vi "TP5.vi"() -> ()   [LabVIEW 2017]
panel:
  out "Boolean 3":bool
  out "Boolean 2":bool
  out "Boolean":bool
  in  "10s":bool
  in  "Tab Control 2":enum32{"Page 1"}(tab)
  in  "Tab Control":enum32{"Page 1"}(tab)
  in  "stop":bool
  in  "pause":bool
  in  "Minuterie":u32 format="%<%M:%S>t"
  in  "rotation":bool
  in  "1m":bool
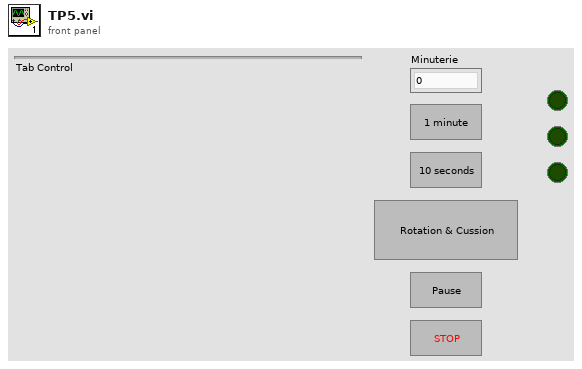
[diagram p1: front panel]
types:
  T1 = enum16{"initialisation", "Mise en marche et vérification", "Cussion", "Pause", "Stop"}
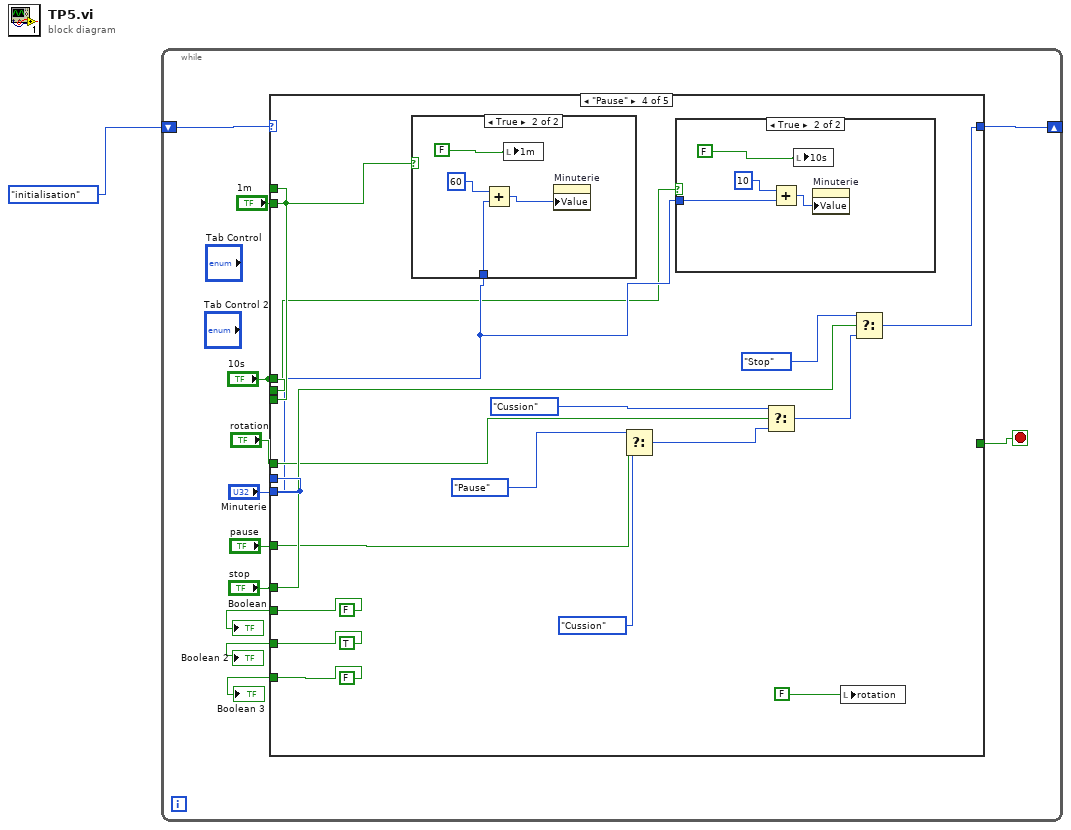
[diagram p0: block diagram]
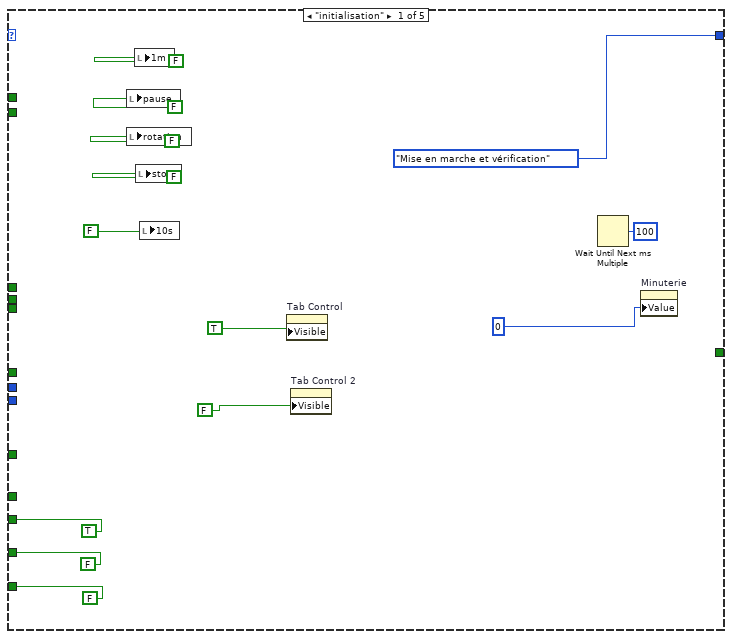
[diagram p2: hidden frame]
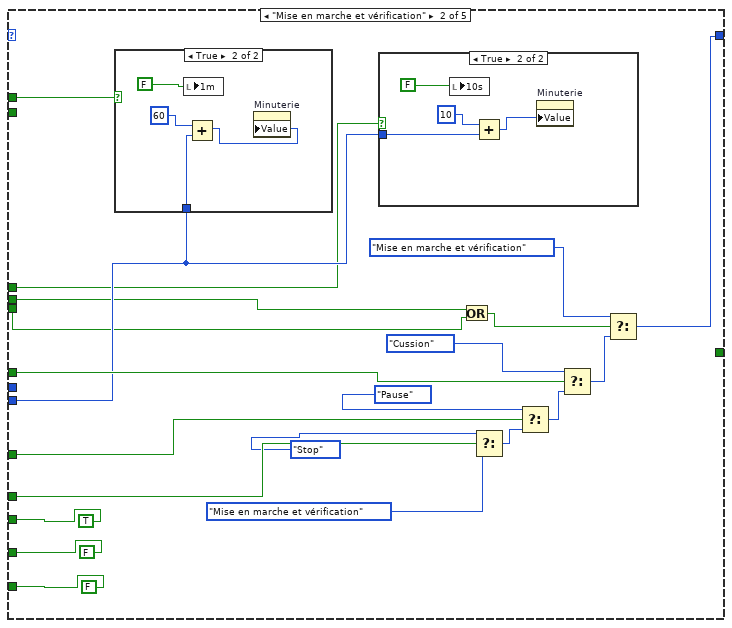
[diagram p3: hidden frame]
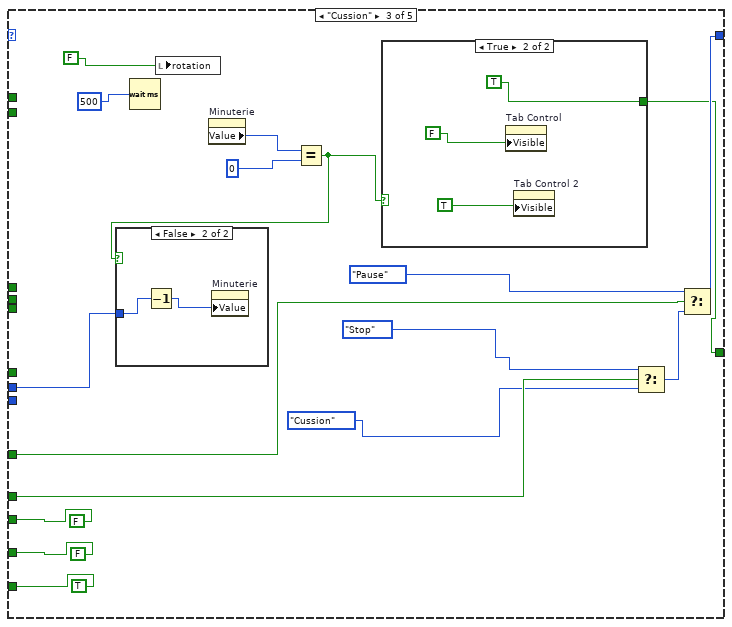
[diagram p6: hidden frame]
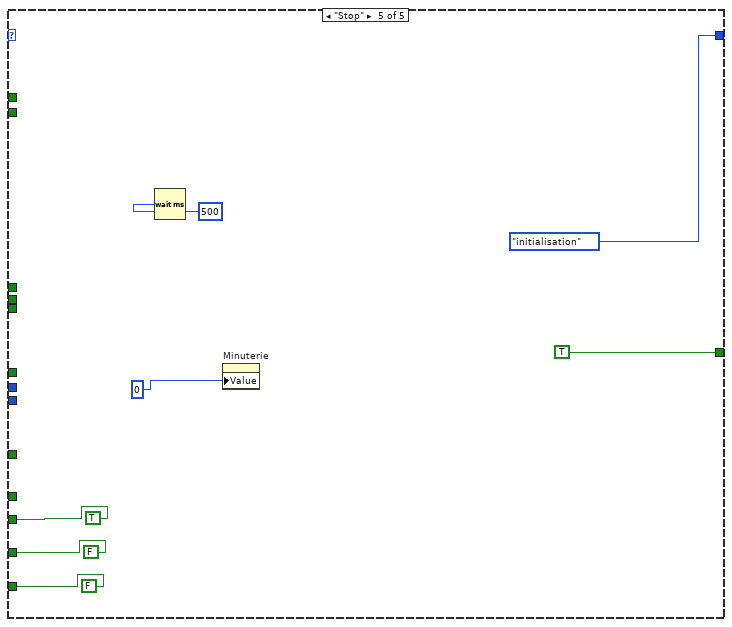
[diagram p11: hidden frame]
diagram:
  n1 = while {
    shift-right: [w12] -> _
    shift-left: T1."initialisation" -> [w13]
    stop <- w11 stop-if-true
    n2 = case shown="\"Pause\"" w13 {
      tunnel: [T1."Mise en marche et vérification" w41 w69 w90 T1."initialisation"] -> w12
      tunnel: [_ _ w61 _ TRUE] -> w11
      tunnel: "stop" -> [_ w40 w67 w89 _]
      tunnel: "pause" -> [_ w39 w68 w88 _]
      tunnel: "rotation" -> [_ w38 _ w81 _]
      tunnel: "1m" -> [_ w31 _ _ _]
      tunnel: "1m" -> [_ w37 _ _ _]
      tunnel: "Minuterie" -> [_ w34 _ w80 _]
      tunnel: "Minuterie" -> [_ _ w60 _ _]
      tunnel: "10s" -> [_ w33 _ w78 _]
      tunnel: "10s" -> [_ w30 _ _ _]
      tunnel: [FALSE FALSE FALSE TRUE FALSE] -> w5
      tunnel: [TRUE TRUE FALSE FALSE TRUE] -> w4
      tunnel: [FALSE FALSE TRUE FALSE FALSE] -> w3
      tunnel: "1m" -> [_ _ _ w79 _]
      frame "initialisation" {
        n3 = local write "pause"(FALSE) -> ()
        n4 = local write "rotation"(FALSE) -> ()
        n5 = local write "1m"(FALSE) -> ()
        n6 = local write "stop"(FALSE) -> ()
        n7 = local write "10s"(FALSE) -> ()
        n8 = property on="Tab Control" class="TabCtl (strict)"("Visible"=TRUE) -> ()  [unwired: 2 in, 2 out]
        n9 = property on="Tab Control 2" class="TabCtl (strict)"("Visible"=FALSE) -> ()  [unwired: 2 in, 2 out]
        n10 = Wait Until Next ms Multiple(millisecond multiple=100) -> ()  [unwired: 1 out]
        n11 = property on="Minuterie" class="DigNum (strict)"("Value"=0) -> ()  [unwired: 2 in, 2 out]
      }
      frame "Mise en marche et vérification" {
        n12 = case shown="True" w37 {
          tunnel: w34 -> [_ w55]
          frame False {
          }
          frame True {
            n13 = local write "1m"(FALSE) -> ()
            n14 = Add(x=60, y=w55) -> (x+y=w53:u32)
            n15 = property on="Minuterie" class="DigNum (strict)"("Value"=w53) -> ()  [unwired: 2 in, 2 out]
          }
        }
        n16 = case shown="True" w33 {
          tunnel: w34 -> [_ w49]
          frame False {
          }
          frame True {
            n17 = local write "10s"(FALSE) -> ()
            n18 = Add(x=10, y=w49) -> (x+y=w50:u32)
            n19 = property on="Minuterie" class="DigNum (strict)"("Value"=w50) -> ()  [unwired: 2 in, 2 out]
          }
        }
        n20 = Or(x=w30, y=w31) -> (x .or. y?=w32:bool)
        n21 = Select(t=T1."Stop", s=w40, f=T1."Mise en marche et vérification") -> (s? t:f=w47:T1)
        n22 = Select(t=T1."Pause", s=w39, f=w47) -> (s? t:f=w46:T1)
        n23 = Select(t=T1."Cussion", s=w38, f=w46) -> (s? t:f=w42:T1)
        n24 = Select(t=T1."Mise en marche et vérification", s=w32, f=w42) -> (s? t:f=w41:T1)
      }
      frame "Cussion" {
        n25 = Wait (ms)(milliseconds to wait=500) -> ()  [unwired: 1 out]
        n26 = local write "rotation"(FALSE) -> ()
        n27 = property on="Minuterie" class="DigNum (strict)"() -> ("Value"=w63:u32)  [unwired: 2 in, 2 out]
        n28 = Equal?(x=w63, y=0) -> (x = y?=w59:bool)
        n29 = case shown="False" w59 {
          tunnel: w60 -> [_ w73]
          frame True {
          }
          frame False {
            n30 = Decrement(x=w73) -> (x-1=w74:u32)
            n31 = property on="Minuterie" class="DigNum (strict)"("Value"=w74) -> ()  [unwired: 2 in, 2 out]
          }
        }
        n32 = case shown="True" w59 {
          tunnel: [_ TRUE] -> w61
          frame False {
          }
          frame True {
            n33 = property on="Tab Control" class="TabCtl (strict)"("Visible"=FALSE) -> ()  [unwired: 2 in, 2 out]
            n34 = property on="Tab Control 2" class="TabCtl (strict)"("Visible"=TRUE) -> ()  [unwired: 2 in, 2 out]
          }
        }
        n35 = Select(t=T1."Stop", s=w67, f=T1."Cussion") -> (s? t:f=w72:T1)
        n36 = Select(t=T1."Pause", s=w68, f=w72) -> (s? t:f=w69:T1)
      }
      frame "Pause" {
        n37 = case shown="True" w79 {
          tunnel: w80 -> [_ w102]
          frame False {
          }
          frame True {
            n38 = Add(x=60, y=w102) -> (x+y=w99:u32)
            n39 = local write "1m"(FALSE) -> ()
            n40 = property on="Minuterie" class="DigNum (strict)"("Value"=w99) -> ()  [unwired: 2 in, 2 out]
          }
        }
        n41 = Select(t=T1."Pause", s=w88, f=T1."Cussion") -> (s? t:f=w93:T1)
        n42 = case shown="True" w78 {
          tunnel: w80 -> [_ w97]
          frame False {
          }
          frame True {
            n43 = Add(x=10, y=w97) -> (x+y=w95:u32)
            n44 = local write "10s"(FALSE) -> ()
            n45 = property on="Minuterie" class="DigNum (strict)"("Value"=w95) -> ()  [unwired: 2 in, 2 out]
          }
        }
        n46 = Select(t=T1."Cussion", s=w81, f=w93) -> (s? t:f=w94:T1)
        n47 = local write "rotation"(FALSE) -> ()
        n48 = Select(t=T1."Stop", s=w89, f=w94) -> (s? t:f=w90:T1)
      }
      frame "Stop" {
        n49 = Wait (ms)(milliseconds to wait=500) -> ()  [unwired: 1 out]
        n50 = property on="Minuterie" class="DigNum (strict)"("Value"=0) -> ()  [unwired: 2 in, 2 out]
      }
    }
    "Boolean" <- w4
    "Boolean 2" <- w5
    "Boolean 3" <- w3
  }
